vi "load_asap_params.vi"(8 "error in":errorcluster, 11 "ASAP params file":path=path "asap_params.xml") -> (0 "error out":errorcluster)   [LabVIEW 2013]
uses:
  <vilib>/Utility/xml.llb/Read From XML File(string).vi
  globals.vi
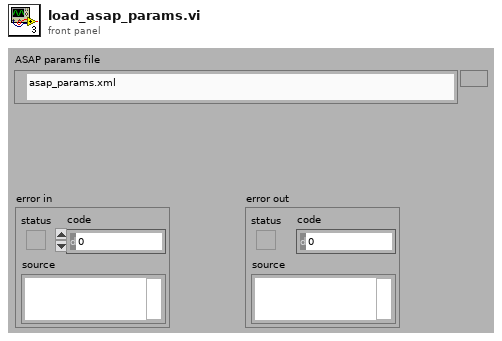
[diagram p1: front panel]
types:
  T1 = cluster{dbl, i32, "Num ASAP channels":i32, "Hardware version":enum16{"ASAP/Trigger", "ASAP/Finder", "ASAP/Micron", "ASAP/Micron 2", "Micron 6DOF"}, "Phase compensation (degrees)":dbl[][], dbl[], "Phase lags (degrees)":dbl[], "Gain calibration":sgl[][]}
  T2 = enum16{"ASAP/Trigger", "ASAP/Finder", "ASAP/Micron", "ASAP/Micron 2", "Micron 6DOF"}
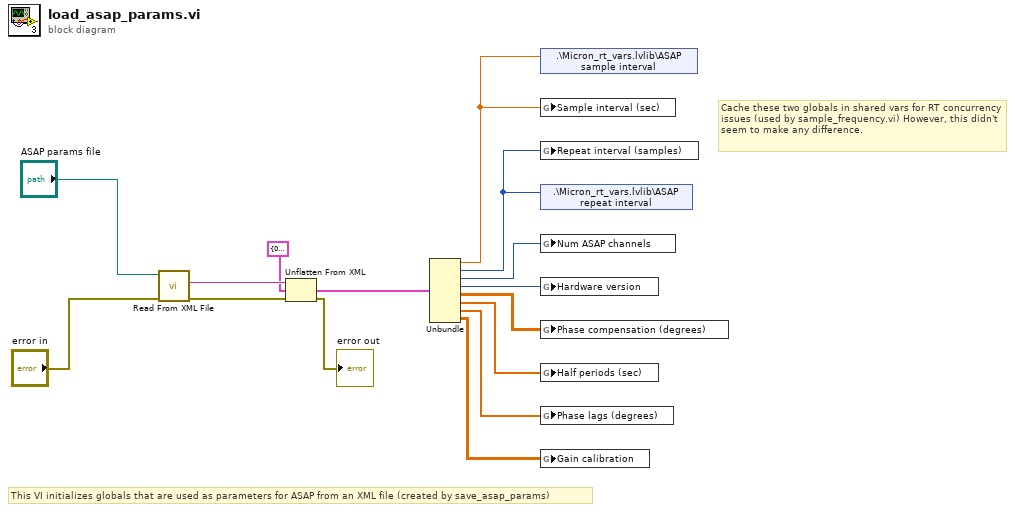
[diagram p0: block diagram]
diagram:
  # "Cache these two globals in shared vars for RT concurrency issues (used by sample_frequency.vi) However, this didn't seem to make any difference."
  # "This VI initializes globals that are used as parameters for ASAP from an XML file (created by save_asap_params)"
  n1 = call-poly <vilib>:"Read From XML File.vi"("error in (no error)"="error in", "XML File Path"="ASAP params file") -> ("error out"=w14:errorcluster, "XML Elements"=w15:string)  [unwired: 8 out]
  n2 = Unflatten From XML(xml string=w15, type=T1 {0.0, 0, "Num ASAP channels"=0, "Hardware version"=enum."ASAP/Trigger", "Phase compensation (degrees)"=[], [], "Phase lags (degrees)"=[], "Gain calibration"=[]} ("output cluster"), error in (no error)=w14) -> (value=w10:T1, error out=→"error out":errorcluster)
  n3 = Unbundle(w10) -> (w4:dbl, w3:i32, "Num ASAP channels"=w9:i32, "Hardware version"=w8:T2, "Phase compensation (degrees)"=w7:dbl[][], w6:dbl[], "Phase lags (degrees)"=w5:dbl[], "Gain calibration"=w1:sgl[][])
  n4 = shared-variable ".\\Micron_rt_vars.lvlib\\ASAP sample interval"(w4) -> ()  [unwired: 1 in, 1 out]
  n5 = global write "globals.vi" "Sample interval (sec)"(w4) -> ()
  n6 = global write "globals.vi" "Repeat interval (samples)"(w3) -> ()
  n7 = shared-variable ".\\Micron_rt_vars.lvlib\\ASAP repeat interval"(w3) -> ()  [unwired: 1 in, 1 out]
  n8 = global write "globals.vi" "Num ASAP channels"(w9) -> ()
  n9 = global write "globals.vi" "Hardware version"(w8) -> ()
  n10 = global write "globals.vi" "Phase compensation (degrees)"(w7) -> ()
  n11 = global write "globals.vi" "Half periods (sec)"(w6) -> ()
  n12 = global write "globals.vi" "Phase lags (degrees)"(w5) -> ()
  n13 = global write "globals.vi" "Gain calibration"(w1) -> ()
